vi "Pipeline 3ch.vi"(10 "data in":T1[](array[typedef]), 11 "data in":T1[](array[typedef])) -> (2 "data out":T1[](array[typedef]), 3 "data out":T1[](array[typedef]))   [LabVIEW 2025, in "niUSRP Rx DSP v2 FPGA.lvclass"]
uses:
  niUSRP Rx DSP v2 FPGA.lvclass
  niUSRP Rx DSP v2 FPGA.lvclass/niUSRP Rx DSP v2 FPGA.ctl
  <instrlib>/_niInstr/DSP/v1/Shared/Public/IQ Data.ctl
  <instrlib>/_niInstr/DSP/v1/Shared/niInstr DSP v1 Shared.lvlib
panel:
  out "data out":T1[](array[typedef])
  in  "data in":T1[](array[typedef])
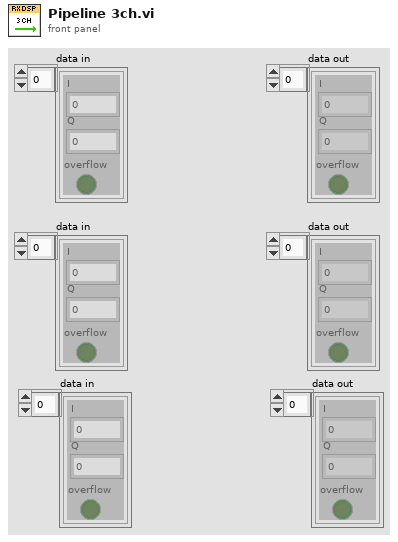
[diagram p1: front panel]
types:
  T1 = typedef "niInstr DSP v1 Shared.lvlib/IQ Data.ctl" = cluster{"I":fxp<+/-,18,1>, "Q":fxp<+/-,18,1>, "overflow":bool}
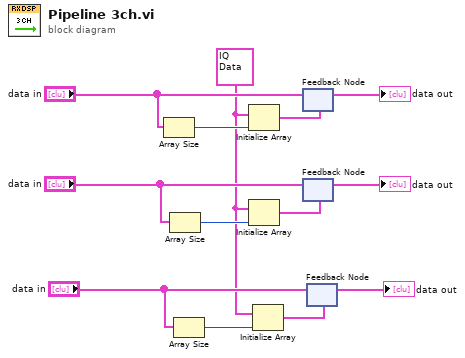
[diagram p0: block diagram]
diagram:
  w1 = T1 {"I"=0.0, "Q"=0.0, "overflow"=FALSE} ("data")
  n1 = Array Size(array="data in") -> (size(s)=w9:i32)
  n2 = Array Size(array="data in") -> (size(s)=w10:i32)
  n3 = Array Size(array="data in") -> (size(s)=w3:i32)
  n4 = Initialize Array(w1, w9) -> (w13:T1[])
  n5 = Initialize Array(w1, w10) -> (w12:T1[])
  n6 = Initialize Array(w1, w3) -> (w5:T1[])
  n7 = feedback #1(w13) -> (→"data out":T1[])
  n8 = feedback-in #1("data in") -> ()
  n9 = feedback #2(w12) -> (→"data out":T1[])
  n10 = feedback-in #2("data in") -> ()
  n11 = feedback #3(w5) -> (→"data out":T1[])
  n12 = feedback-in #3("data in") -> ()
